vi "Generated Descriptors.vi"() -> (3 "Descriptor Strings":string[](array[string]))   [LabVIEW 2019, in "Service Template.lvlib"]
uses:
  Service Template.lvlib
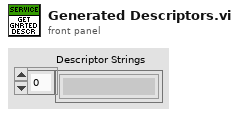
[diagram p1: front panel]
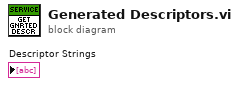
[diagram p0: block diagram]
diagram:
